vi "g_temperature.vi"() -> ()   [LabVIEW 2015]
panel:
  in  "Temperature":dbl
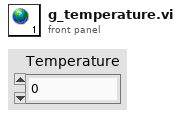
[diagram p1: front panel]
diagram:
